vi "GetPredecessors.vi"(8 "error in (no error)":errorcluster, 10 "NodeReference":refnum<data-value>, 11 "WorldMap in":refnum<class "NI_Robotics_AbstractWorldMap.lvclass">) -> (0 "error out":errorcluster, 1 "EdgeCost":dbl[](array[numeric]), 2 "Predecessors":refnum<data-value>[](array[refnum]), 3 "WorldMap out":refnum<class "NI_Robotics_AbstractWorldMap.lvclass">)   [LabVIEW 2017, in "NI_Robotics_AbstractWorldMap.lvclass"]
uses:
  <vilib>/robotics/Navigation/shared/WorldMap/AbstractWorldMap/NI_Robotics_AbstractWorldMap.lvclass
  <vilib>/robotics/Navigation/shared/MapNode/AbstractMapNode/NI_Robotics_AbstractMapNode.lvclass
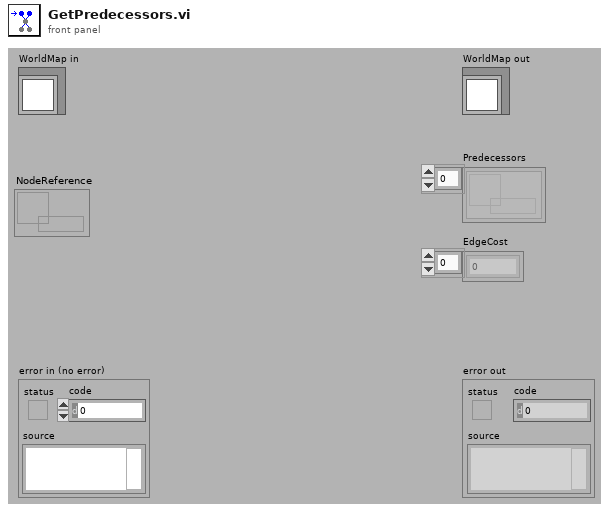
[diagram p1: front panel]
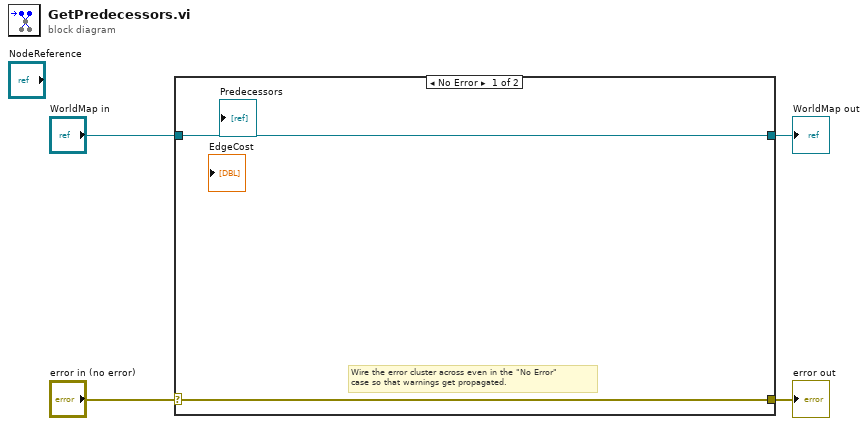
[diagram p0: block diagram]
diagram:
  n1 = case shown="No Error" "error in (no error)" {
    selector: "error in (no error)" -> [w5 w8]
    tunnel: [w5 w8] -> w3
    tunnel: [w6 w7] -> w1
    tunnel: "WorldMap in" -> [w6 w7]
    frame No Error {
      # "Wire the error cluster across even in the \"No Error\"\ncase so that warnings get propagated."
    }
    frame Error {
    }
  }
  "error out" <- w3
  "WorldMap out" <- w1
